vi "PC Benchmarking.vi"() -> ()   [LabVIEW 2013]
doc: "This application launches and executes the Tag Bus Data framework configuration for the specified target alias. This is a simple example of the framework API functions, but may also be a suitable starting point for a Host UI or Thick Client that is running a local version of the framework."
uses:
  <vilib>/NI/Module Execution Interface/Engine Runtime/Execution States.ctl
  <vilib>/NI/Module Execution Interface/Engine Runtime/Fault.ctl
  <vilib>/NI/Tag Bus Module Framework/runtime/error classification.ctl
  <vilib>/NI/Module Execution Interface/Engine Runtime/Engine Runtime Interface.lvclass
  <vilib>/NI/Current Value Table/DataTypes/Double_Read.vi
  <vilib>/NI/Current Value Table/Type to Enum.vi
  <vilib>/NI/Current Value Table/DataTypes/Double_Type To Enum.vi
  <vilib>/NI/Current Value Table/FGVs/CVT Globals.vi
  <vilib>/NI/Current Value Table/FGVs/Tag Memory.vi
  <vilib>/NI/Current Value Table/Memory Block.vi
  <vilib>/NI/Current Value Table/DataTypes/Double_Memory Block.vi
  <vilib>/userdefined/High Color/nirio_resource_hc.ctl
  <vilib>/NI/DCAF/Tag Editor Core/Framework Configuration Classes/target runtime/PL_Target Runtime.lvclass
  <vilib>/NI/Tag Bus Module Framework/FPGA manager/FPGA manager.lvlib
  <vilib>/rvi/interface/nirviOpenFPGA/nirviOpenFPGA.xnode
  <vilib>/NI/Tag Bus Module Framework/FPGA manager/methods.ctl
  <vilib>/NI/Current Value Table/Current Value Table.lvlib
  <vilib>/NI/Tag Bus Module Framework/runtime/TBM module execution interface.lvclass
panel:
  out "Scaled Double":dbl
  out "Double":dbl
  in  "configuration file path":path=path "C:/Users/bsnover/Desktop/DCAF Integration Testing/Testing Project/Integration Testing Configuration.pcfg"
  in  "target alias":string="PC Benchmarking"
  out "engine status":T4(array[cluster])
  in  "stop":bool
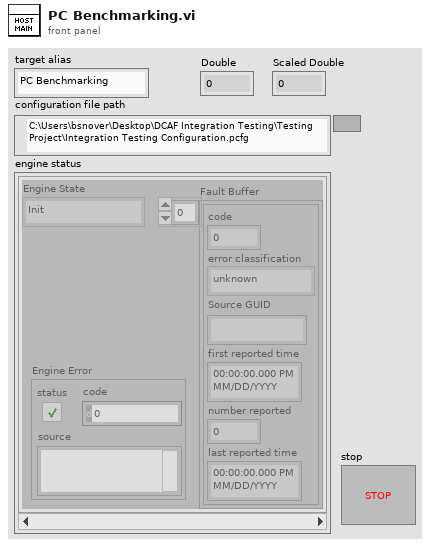
[diagram p1: front panel]
types:
  T1 = typedef "Engine Runtime Interface.lvclass/Execution States.ctl" = enum16{"Init", "Pre-Operational", "Safe-Operational", "Operational", "Stopped"}
  T2 = typedef "Engine Runtime Interface.lvclass/Fault.ctl" = cluster{"code":i32, "error classification":T3, "Source GUID":string, "first reported time":timestamp, "number reported":u32, "last reported time":timestamp}
  T3 = typedef "TBM module execution interface.lvclass/error classification.ctl" = enum16{"unknown", "none", "trivial", "recoverable", "critical"}
  T4 = cluster{"Engine State":T1, "Fault Buffer":T2[], "Engine Error":errorcluster}[]
  T5 = typedef "FPGA manager.lvlib/methods.ctl" = enum16{"initialize bitfile", "cache bitfile", "locate bitfile", "close bitfile", "clear manager"}
  T6 = typedef "nirio_resource_hc.ctl" = tag
  T7 = cluster{"Engine State":T1, "faults":T2[], "Engine Error":errorcluster}
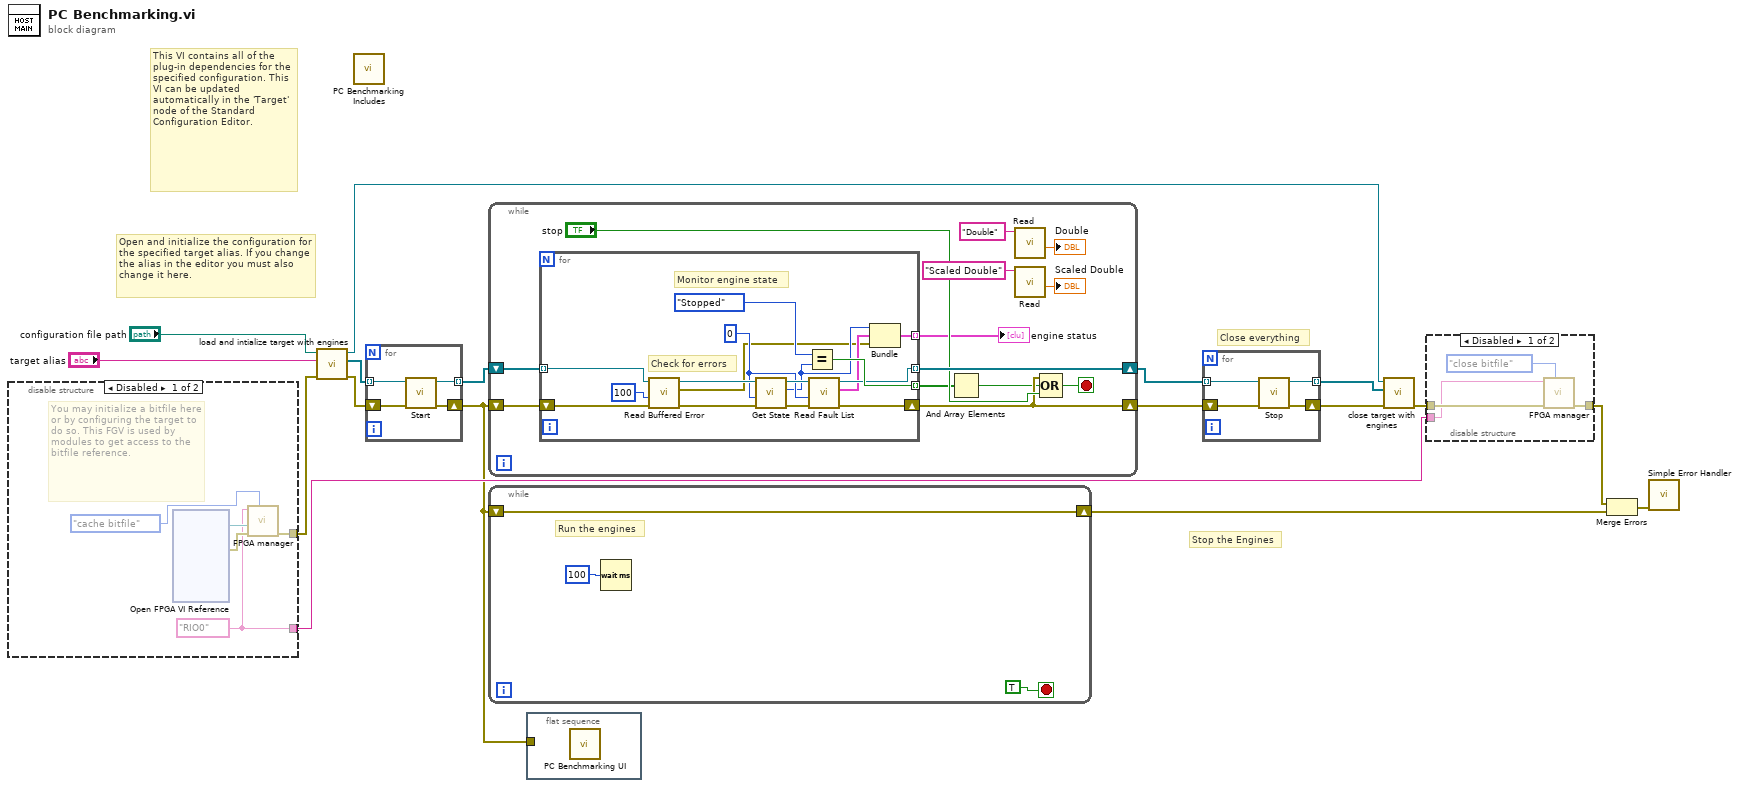
[diagram p0: block diagram]
diagram:
  # "Open and initialize the configuration for the specified target alias. If you change the alias in the editor you must also change it here."
  # "Close everything"
  # "Stop the Engines"
  # "This VI contains all of the plug-in dependencies for the specified configuration. This VI can be updated automatically in the 'Target' node of the Standard Configuration Editor."
  # "Run the engines"
  n1 = disable-structure shown="Disabled" {
    disable-tunnel: [w22 _] -> w7
    disable-tunnel: [w18 _] -> w6
    frame Disabled {
      w18 = T6 "RIO0" ("RIO resource")
      # "You may initialize a bitfile here or by configuring the target to do so. This FGV is used by modules to get access to the bitfile reference."
      n2 = xnode "Open FPGA VI Reference"() -> ("FPGA VI Reference Out"=w20:refnum<k20>, "error out"=w21:errorcluster)  [unwired: 2 in]
      n3 = call <vilib>:"FPGA manager.vi"("action"=methods."cache bitfile", "error in"=w21, "bitfile to cache"=w20, "RIO resource"=w18) -> ("error out"=w22:errorcluster)  [unwired: 5 in, 2 out]
    }
    frame Enabled {
    }
  }
  n4 = call <vilib>:"load and intialize target with engines.vi"("error in"=w7, "target alias"="target alias", "file path"="configuration file path") -> ("error out"=w14:errorcluster, "engine runtime interfaces"=w13:refnum<class "Engine Runtime Interface.lvclass">[], "target runtime"=w10:refnum<class "PL_Target Runtime.lvclass">)  [unwired: 6 in]
  n5 = call "PC Benchmarking Includes.vi"() -> ()  [unwired: 12 in]
  n6 = for {
    tunnel: [w26] -> w17 mode=indexing
    tunnel: w13 -> [w23] mode=indexing
    shift-right: [w25] -> w1
    shift-left: w14 -> [w24]
    n7 = call-dynamic "Start.vi"("error in"=w24, "Engine Runtime Interface in"=w23) -> ("error out"=w25:errorcluster, "Engine Runtime Interface out"=w26:refnum<class "Engine Runtime Interface.lvclass">)  [unwired: 8 in]
  }
  n8 = while {
    shift-right: [w37] -> w16
    shift-left: w17 -> [w39]
    shift-right: [w34] -> w15
    shift-left: w1 -> [w38]
    stop <- w35 stop-if-true
    n9 = for {
      tunnel: w39 -> [w55] mode=indexing
      tunnel: [w46] -> w37 mode=indexing
      tunnel: [w50] -> w32 mode=indexing
      shift-right: [w45] -> w34
      shift-left: w38 -> [w54]
      tunnel: [w40] -> w33 mode=indexing
      w44 = 0 ("timeout (-1)")
      # "Monitor engine state"
      # "Check for errors"
      n10 = call-dynamic "Read Buffered Error.vi"("error in"=w54, "timeout in ms (0)"=100, "Engine Runtime Interface in"=w55) -> ("error out"=w52:errorcluster, "Engine Error"=w41:errorcluster, "Engine Runtime Interface out"=w53:refnum<class "Engine Runtime Interface.lvclass">)  [unwired: 6 in]
      n11 = call-dynamic "Get State.vi"("error in"=w52, "timeout (-1)"=w44, "Engine Runtime Interface in"=w53) -> ("error out"=w48:errorcluster, "Engine State"=w43:T1, "Engine Runtime Interface out"=w47:refnum<class "Engine Runtime Interface.lvclass">)  [unwired: 6 in]
      n12 = Equal?(x=Execution_States."Stopped" ("Engine State"), y=w43) -> (x = y?=w50:bool)
      n13 = call-dynamic "Read Fault List.vi"("error in"=w48, "timeout (-1)"=w44, "Engine Runtime Interface in"=w47) -> ("error out"=w45:errorcluster, "faults"=w42:T2[], "Engine Runtime Interface out"=w46:refnum<class "Engine Runtime Interface.lvclass">)  [unwired: 6 in]
      n14 = Bundle("Engine State"=w43, "faults"=w42, "Engine Error"=w41) -> (w40:T7)  [unwired: 1 in]
    }
    "engine status" <- w33
    n15 = And Array Elements(Boolean array=w32) -> (logical AND=w31:bool)
    n16 = call-poly <vilib>:"Read.vi"("Tag Name"="Double") -> ("Value"=→"Double":dbl)  [unwired: 9 in, 1 out]
    n17 = call-poly <vilib>:"Read.vi"("Tag Name"="Scaled Double") -> ("Value"=→"Scaled Double":dbl)  [unwired: 9 in, 1 out]
    n18 = Compound Arithmetic op=OR(w34, w31, "stop") -> (w35:bool)
  }
  n19 = while {
    shift-right: [w56] -> w5
    shift-left: w1 -> [w56]
    stop <- TRUE stop-if-true
    n20 = Wait (ms)(milliseconds to wait=u32 100) -> ()  [unwired: 1 out]
  }
  n21 = flat-sequence {
    tunnel: w1 -> [_]
    frame #0 {
      n22 = call "PC Benchmarking UI.vi"() -> ()  [unwired: 12 in]
    }
  }
  n23 = for {
    tunnel: w16 -> [w62] mode=indexing
    shift-right: [w59] -> w9
    shift-left: w15 -> [w61]
    tunnel: [w60] -> w11 mode=indexing
    n24 = call-dynamic "Stop.vi"("error in"=w61, "Engine Runtime Interface in"=w62) -> ("error out"=w59:errorcluster, "Engine Runtime Interface out"=w60:refnum<class "Engine Runtime Interface.lvclass">)  [unwired: 8 in]
  }
  n25 = call <vilib>:"close target with engines.vi"("error in"=w9, "Engine Runtime Interfaces"=w11, "Target Runtime"=w10) -> ("error out"=w4:errorcluster)  [unwired: 8 in]
  n26 = disable-structure shown="Disabled" {
    disable-tunnel: [w65 w67] -> w3
    disable-tunnel: w4 -> [w66 w67]
    disable-tunnel: w6 -> [w63 _]
    frame Disabled {
      n27 = call <vilib>:"FPGA manager.vi"("action"=methods."close bitfile", "error in"=w66, "RIO resource"=w63) -> ("error out"=w65:errorcluster)  [unwired: 6 in, 2 out]
    }
    frame Enabled {
    }
  }
  n28 = Merge Errors(w3, w5) -> (w2:errorcluster)
  n29 = call <vilib>:"Simple Error Handler.vi"("error in (no error)"=w2) -> ()  [unwired: 4 in, 5 out]
